vi "Post-Install Custom Action.vi"(10 "Variant":variant) -> (0 "error out":errorcluster)   [LabVIEW 2020]
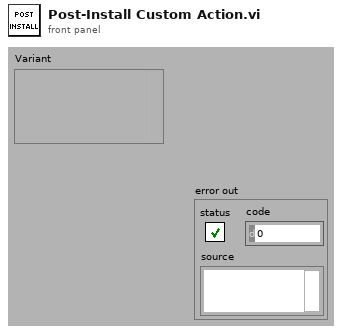
[diagram p1: front panel]
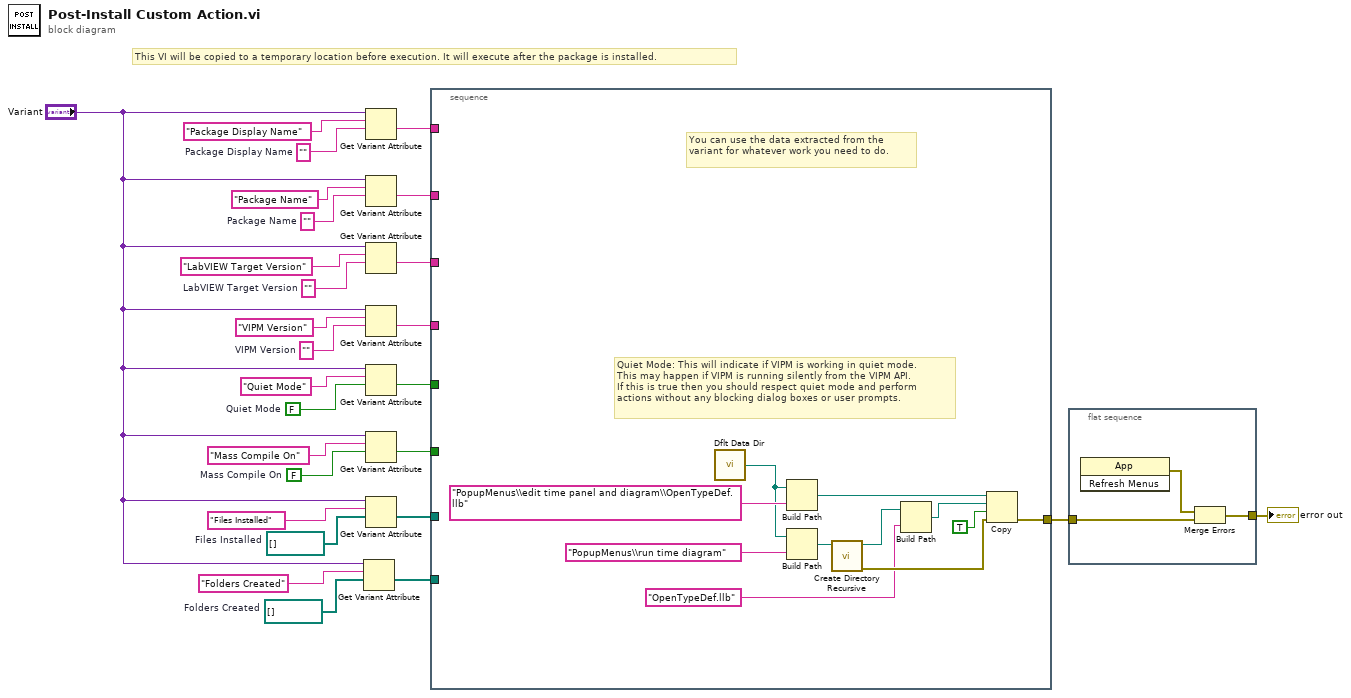
[diagram p0: block diagram]
diagram:
  w3 = path[] []  # Folders Created
  w4 = path[] []  # Files Installed
  w10 = FALSE  # Mass Compile On
  w11 = ""  # Package Display Name
  w18 = FALSE  # Quiet Mode
  w21 = ""  # VIPM Version
  w23 = ""  # LabVIEW Target Version
  w25 = ""  # Package Name
  # "This VI will be copied to a temporary location before execution. It will execute after the package is installed."
  n1 = Get Variant Attribute(Variant="Variant", name="Folders Created", default value (empty Variant)=w3) -> (value=w8:path[])  [unwired: 1 in, 3 out]
  n2 = Get Variant Attribute(Variant="Variant", name="Package Display Name", default value (empty Variant)=w11) -> (value=w17:string)  [unwired: 1 in, 3 out]
  n3 = Get Variant Attribute(Variant="Variant", name="Package Name", default value (empty Variant)=w25) -> (value=w16:string)  [unwired: 1 in, 3 out]
  n4 = Get Variant Attribute(Variant="Variant", name="LabVIEW Target Version", default value (empty Variant)=w23) -> (value=w15:string)  [unwired: 1 in, 3 out]
  n5 = Get Variant Attribute(Variant="Variant", name="VIPM Version", default value (empty Variant)=w21) -> (value=w14:string)  [unwired: 1 in, 3 out]
  n6 = Get Variant Attribute(Variant="Variant", name="Quiet Mode", default value (empty Variant)=w18) -> (value=w13:bool)  [unwired: 1 in, 3 out]
  n7 = Get Variant Attribute(Variant="Variant", name="Mass Compile On", default value (empty Variant)=w10) -> (value=w12:bool)  [unwired: 1 in, 3 out]
  n8 = Get Variant Attribute(Variant="Variant", name="Files Installed", default value (empty Variant)=w4) -> (value=w7:path[])  [unwired: 1 in, 3 out]
  n9 = stacked-sequence {
    tunnel: w17 -> [_]
    tunnel: w16 -> [_]
    tunnel: w15 -> [_]
    tunnel: w14 -> [_]
    tunnel: w13 -> [_]
    tunnel: w12 -> [_]
    tunnel: w7 -> [_]
    tunnel: w8 -> [_]
    tunnel: [w38] -> w2
    frame #0 {
      # "Quiet Mode: This will indicate if VIPM is working in quiet mode.\nThis may happen if VIPM is running silently from the VIPM API.\nIf this is true then you should respect quiet mode and perform\nactions without any blocking dialog boxes or user prompts."
      # "You can use the data extracted from the variant for whatever work you need to do."
      n10 = call <vilib>:"Dflt Data Dir.vi"() -> ("App:Default Data Directory"=w34:path)
      n11 = Build Path(base path=w34, name or relative path="PopupMenus\\edit time panel and diagram\\OpenTypeDef.llb") -> (appended path=w28:path)
      n12 = Build Path(base path=w34, name or relative path="PopupMenus\\run time diagram") -> (appended path=w32:path)
      n13 = call <vilib>:"Create Directory Recursive.vi"("directory"=w32) -> ("error out"=w36:errorcluster, "directory copy"=w31:path)  [unwired: 4 in, 1 out]
      n14 = Build Path(base path=w31, name or relative path="OpenTypeDef.llb") -> (appended path=w29:path)
      n15 = Copy(8:w36, 9:TRUE, 10:w29, 11:w28) -> (0:w38:errorcluster)  [unwired: 1 in, 2 out]
    }
  }
  n16 = flat-sequence {
    tunnel: w2 -> [w41]
    tunnel: [w39] -> w1
    frame #0 {
      n17 = invoke class="App" method="Refresh Menus"() -> (error out=w40:errorcluster)  [unwired: 3 in, 2 out]
      n18 = Merge Errors(w40, w41) -> (w39:errorcluster)
    }
  }
  "error out" <- w1
